vi "Build Coincidence.vi"(0 "Coincs in":T2[](array[typedef]), 5 "Secondary hit in":T1, 7 "Primary hit in":T1, 9 "Primary ID":i8, 11 "Secondary ID":i8, 12 "Primary true hit time":u64, 13 "Secondary true hit time":u64) -> (4 "Coincs out":T2[](array[typedef]), 6 "Secondary hit out":T1, 10 "Primary hit out":T1, 14 "secondary counted as coinc":bool, 15 "Primary counted as coinc":bool)   [LabVIEW 2016]
uses:
  Typedefs/Coincidence.ctl
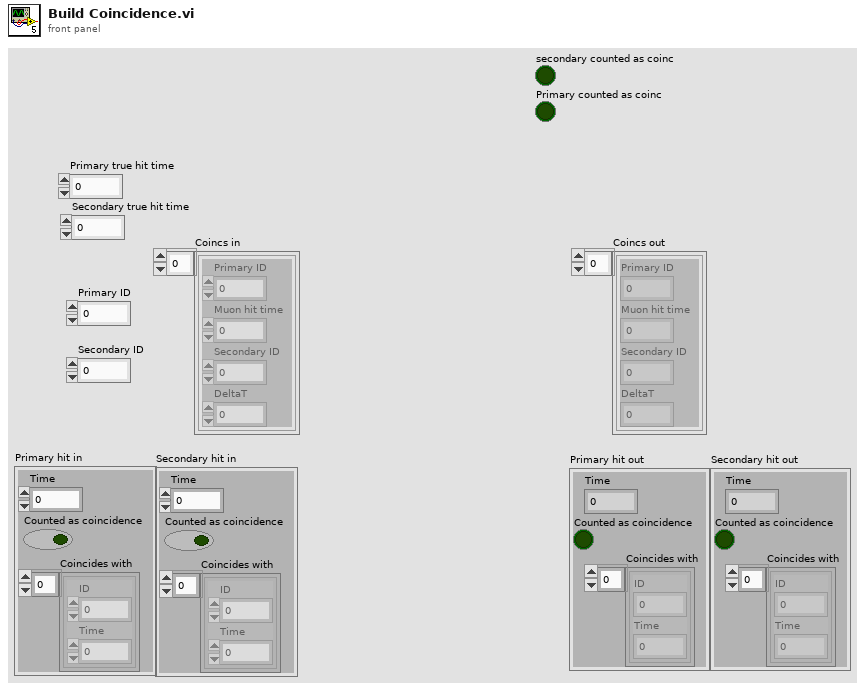
[diagram p1: front panel]
types:
  T1 = cluster{"Time":u64, "Counted as coincidence":bool, "Coincides with":cluster{"ID":i8, "Time":u64}[]}
  T2 = typedef "Coincidence.ctl" = cluster{"Primary ID":i8, "Muon hit time":u64, "Secondary ID":i8, "DeltaT":i32}
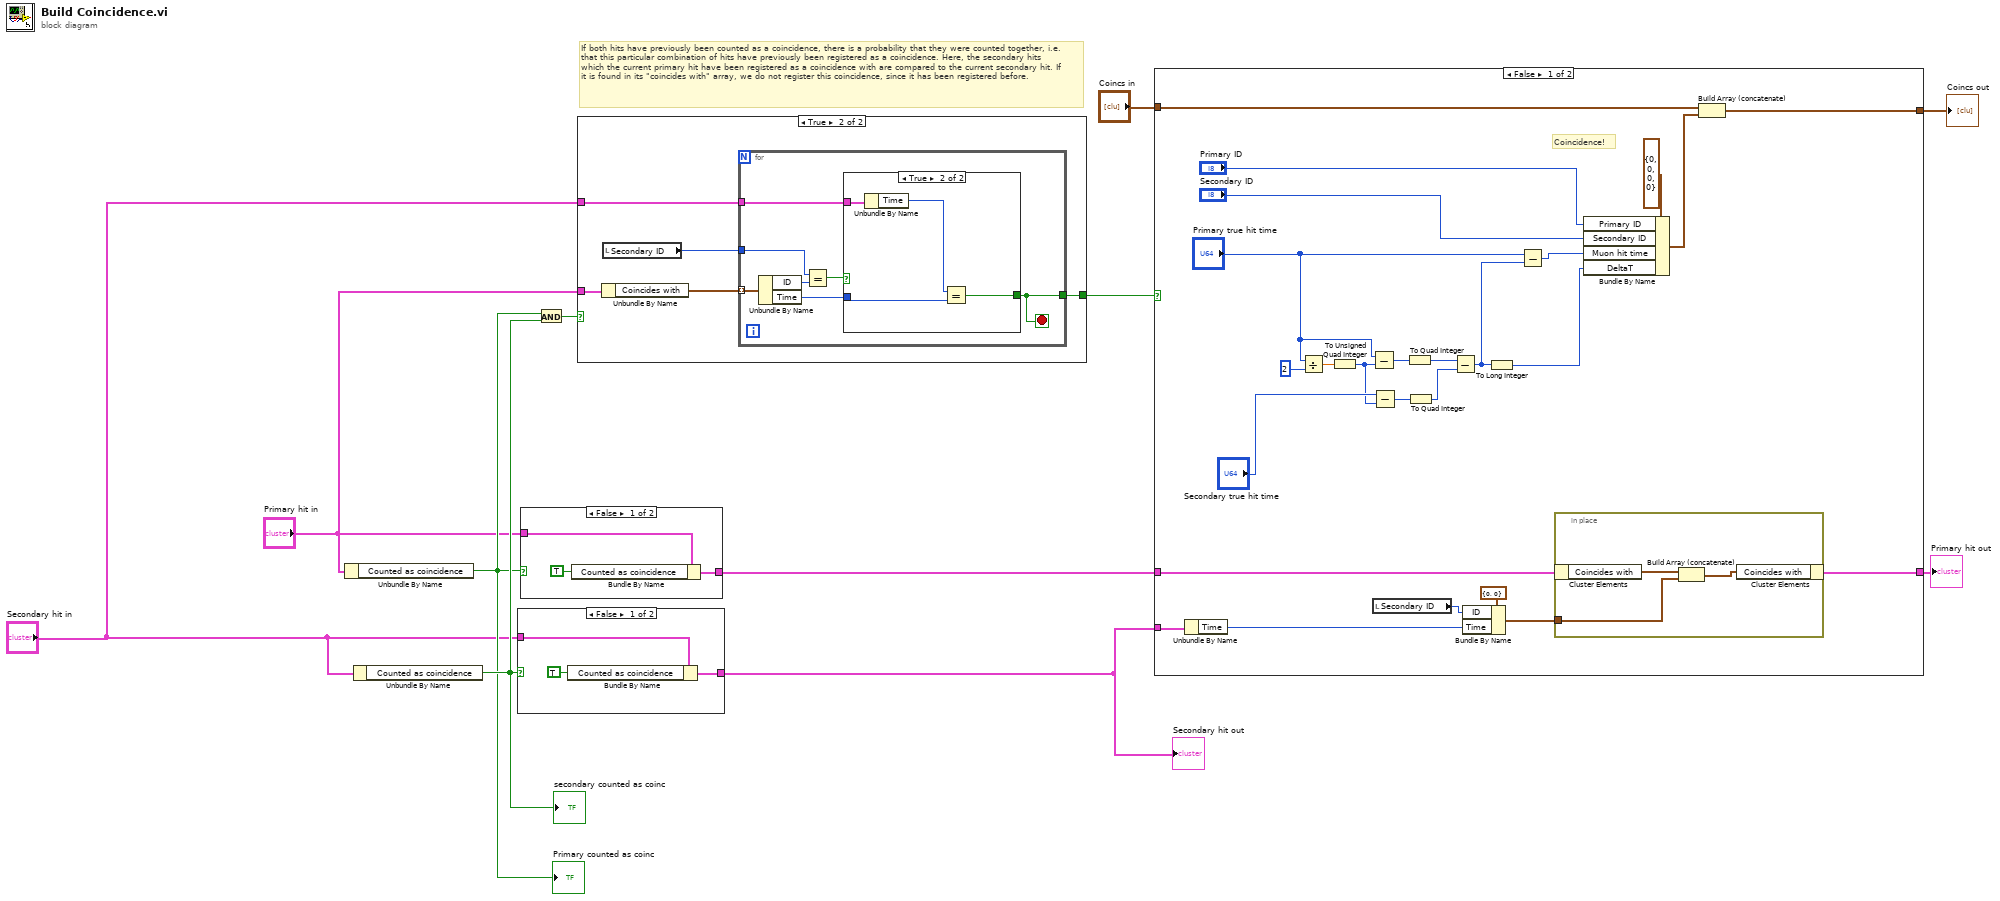
[diagram p0: block diagram]
diagram:
  # "If both hits have previously been counted as a coincidence, there is a probability that they were counted together, i.e. that this particular combination of hits have previously been registered as a coincidence. Here, the secondary hits which the current primary hit have been registered as a coincidence with are compared to the current secondary hit. If it is found in its \"coincides with\" array, we do not register this coincidence, since it has been registered before."
  n1 = Unbundle By Name("Primary hit in") -> ("Counted as coincidence"=w10:bool)
  "Primary counted as coinc" <- w10
  n2 = Unbundle By Name("Secondary hit in") -> ("Counted as coincidence"=w11:bool)
  "secondary counted as coinc" <- w11
  n3 = case shown="False" w11 {
    tunnel: "Secondary hit in" -> [w14 w15]
    tunnel: [w12 w15] -> w4
    frame False {
      n4 = Bundle By Name(cluster=w14, "Counted as coincidence"=TRUE) -> (w12:T1)
    }
    frame True {
    }
  }
  "Secondary hit out" <- w4
  n5 = case shown="False" w10 {
    tunnel: "Primary hit in" -> [w18 w19]
    tunnel: [w16 w19] -> w5
    frame False {
      n6 = Bundle By Name(cluster=w18, "Counted as coincidence"=TRUE) -> (w16:T1)
    }
    frame True {
    }
  }
  n7 = And(x=w10, y=w11) -> (x .and. y?=w9:bool)
  n8 = case shown="True" w9 {
    tunnel: "Primary hit in" -> [_ w24]
    tunnel: "Secondary hit in" -> [_ w21]
    tunnel: [_ w20] -> w6
    frame False {
    }
    frame True {
      n9 = Unbundle By Name(w24) -> ("Coincides with"=w23:cluster{"ID":i8, "Time":u64}[])
      n10 = local read "Secondary ID"() -> (w22:i8)
      n11 = for {
        tunnel: w23 -> [w31] mode=indexing
        tunnel: w22 -> [w29]
        tunnel: w21 -> [w26]
        tunnel: [w25] -> w20
        stop <- w25 stop-if-true
        n12 = Unbundle By Name(w31) -> ("ID"=w30:i8, "Time"=w27:u64)
        n13 = Equal?(x=w29, y=w30) -> (x = y?=w28:bool)
        n14 = case shown="True" w28 {
          tunnel: w27 -> [_ w34]
          tunnel: w26 -> [_ w35]
          tunnel: [_ w32] -> w25
          frame False {
          }
          frame True {
            n15 = Unbundle By Name(w35) -> ("Time"=w33:u64)
            n16 = Equal?(x=w33, y=w34) -> (x = y?=w32:bool)
          }
        }
      }
    }
  }
  n17 = case shown="False" w6 {
    tunnel: w5 -> [w53 w64]
    tunnel: w4 -> [w56 _]
    tunnel: [w54 w64] -> w1
    tunnel: [w49 w65] -> w3
    tunnel: "Coincs in" -> [w48 w65]
    frame False {
      # "Coincidence!"
      n18 = Unbundle By Name(w56) -> ("Time"=w50:u64)
      n19 = Divide(x="Primary true hit time", y=u64 2) -> (x/y=w47:dbl)
      n20 = To Unsigned Quad Integer(1:w47) -> (0:w43:u64)
      n21 = Subtract(x="Primary true hit time", y=w43) -> (x-y=w42:u64)
      n22 = Subtract(x="Secondary true hit time", y=w43) -> (x-y=w41:u64)
      n23 = local read "Secondary ID"() -> (w52:i8)
      n24 = To Quad Integer(1:w42) -> (0:w40:i64)
      n25 = To Quad Integer(1:w41) -> (0:w39:i64)
      n26 = Subtract(x=w40, y=w39) -> (x-y=w37:i64)
      n27 = Bundle By Name(cluster=cluster{"ID":i8, "Time":u64} {"ID"=0, "Time"=0} ("coinc hit"), "ID"=w52, "Time"=w50) -> (w55:cluster{"ID":i8, "Time":u64})
      n28 = To Long Integer(number=w37) -> (32bit integer=w38:i32)
      n29 = Subtract(x="Primary true hit time", y=w37) -> (x-y=w46:u64)
      n30 = in-place {
        in-place-border: w55 -> [w62]
        n31 = in-place-cluster #1(w53) -> ("Coincides with"=w63:cluster{"ID":i8, "Time":u64}[])
        n32 = Build Array (concatenate)(w63, w62) -> (w61:cluster{"ID":i8, "Time":u64}[])
        n33 = in-place-cluster #1("Coincides with"=w61) -> (w54:T1)
      }
      n34 = Bundle By Name(cluster=T2 {"Primary ID"=0, "Muon hit time"=0, "Secondary ID"=0, "DeltaT"=0} ("Coincidence"), "Primary ID"="Primary ID", "Secondary ID"="Secondary ID", "Muon hit time"=w46, "DeltaT"=w38) -> (w59:T2)
      n35 = Build Array (concatenate)(w48, w59) -> (w49:T2[])
    }
    frame True {
    }
  }
  "Coincs out" <- w3
  "Primary hit out" <- w1
